vi "Command-RegisterWindow.vi"(8 "error in (no error)":errorcluster, 10 "Data":T1, 11 "Engine in":refnum<class "Engine.lvclass">) -> (0 "error out":errorcluster, 3 "Engine out":refnum<class "Engine.lvclass">)   [LabVIEW 2024, in "GLF.lvlib" / "Engine.lvclass"]
uses:
  Engine.lvclass
  Engine.lvclass/Engine.ctl
  Window/Window.lvclass
  Command-RegisterWindow--cluster.ctl
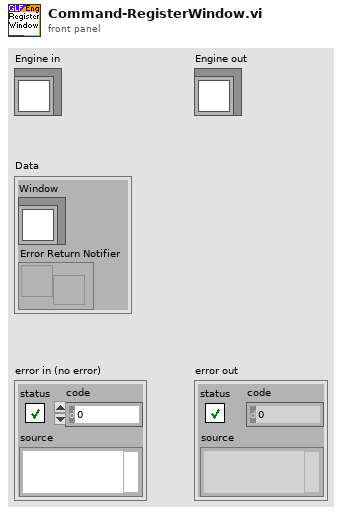
[diagram p1: front panel]
types:
  T1 = typedef "GLF.lvlib/Engine.lvclass/Command-RegisterWindow--cluster.ctl" = cluster{"Window":refnum<class "Window.lvclass">, "Error Return Notifier":refnum<notifier>}
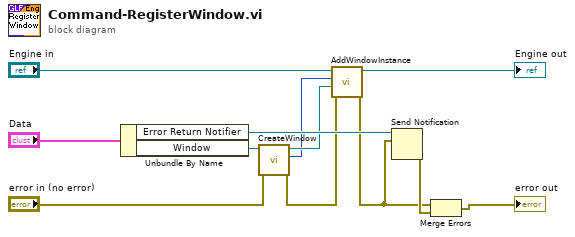
[diagram p0: block diagram]
diagram:
  n1 = Unbundle By Name("Data") -> ("Error Return Notifier"=w12:refnum<notifier>, "Window"=w10:refnum<class "Window.lvclass">)
  n2 = call "CreateWindow.vi"("error in (no error)"="error in (no error)", "Window in"=w10) -> ("error out"=w6:errorcluster, "Window [SDL_Window *]"=w7:i64, "Window out"=w9:refnum<class "Window.lvclass">)  [unwired: 7 in]
  n3 = call "AddWindowInstance.vi"("error in (no error)"=w6, "Window Instance"=w9, "SDL_Window *"=w7, "Engine in"="Engine in") -> ("error out"=w8:errorcluster, "Engine out"=→"Engine out":refnum<class "Engine.lvclass">)  [unwired: 6 in]
  n4 = Send Notification(notification=w8, notifier=w12) -> (error out=w11:errorcluster)  [unwired: 1 in, 1 out]
  n5 = Merge Errors(w8, w11) -> (→"error out":errorcluster)
